vi "Measurement Logic.vi"() -> ()   [LabVIEW 2021, in "audio_acMeasurement.lvlib"]
uses:
  audio_acMeasurement.lvlib
  Measurement Configuration.ctl
  <vilib>/MeasurementLink/MeasurementLink Measurement Server/Classes/MeasurementContext/MeasurementContext.lvclass
  Measurement Results.ctl
  <vilib>/PDM Acquisition Toolkit/host/Classes/Tasks/PCM Input/Controls/DVR PCM Input Task.ctl
  <vilib>/PDM Acquisition Toolkit/host/Classes/Tasks/PCM Input/PCM Input Task.lvclass
  shared/controls/Protocol settings.ctl
  <vilib>/DAQmx/create/channels.llb/DAQmx Create Channel (AO-Voltage-Basic).vi
  <vilib>/DAQmx/configure/timing.llb/DAQmx Timing (Sample Clock).vi
  <vilib>/DAQmx/create/channels.llb/DAQmx Create Channel (AO-FuncGen).vi
  <vilib>/PDM Acquisition Toolkit/host/API/Public/Start/Start PCM Input Task.vi
  <vilib>/PDM Acquisition Toolkit/host/API/Public/Read/Read PCM Input Waveform.vi
  <vilib>/PDM Acquisition Toolkit/host/API/Public/Clear/Clear PCM Input Task.vi
  <resource>/objmgr/daqmx.rc
  <vilib>/PDM Acquisition Toolkit/host/API/PDM Acquisition Toolkit.lvlib
panel:
  out "Measurement Results":T1
  out "Measurement Context out":refnum<class "MeasurementContext.lvclass">
  in  "Measurement Context":refnum<class "MeasurementContext.lvclass">
  in  "Measurement Configuration":T2={"Band start"=20.0, "Band stop"=20000.0, "Weighting filter"=0, "Full scale range"=3.16, "Channel name"="0L", "Analog source resource name"="", "Frequency"=1000.0, "Amplitude"=1.0, "Protocol capture resource name"="", "Data line"=0, "Channel"=0, "Clock rate"=12288000, "Number of words"=19200, "Sensitivity"=0.34762} {"Data line" format="%#.0f"}
  out "error out":errorcluster
  in  "error in":errorcluster
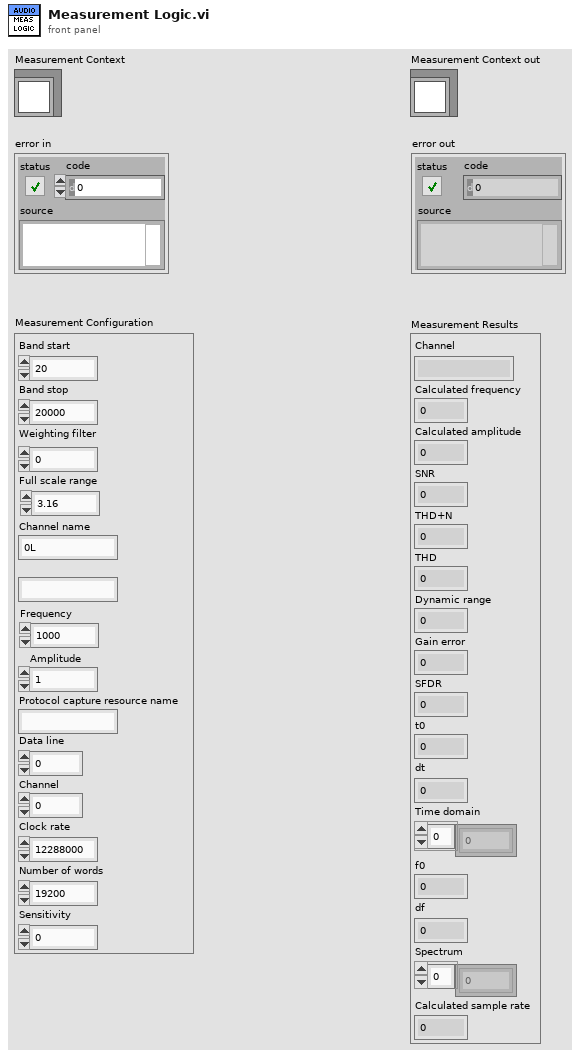
[diagram p1: front panel]
types:
  T1 = typedef "audio_acMeasurement.lvlib/Measurement Results.ctl" = cluster{"Channel":string, "Calculated frequency":dbl, "Calculated amplitude":dbl, "SNR":dbl, "THD+N":dbl, "THD":dbl, "Dynamic range":dbl, "Gain error":dbl, "SFDR":dbl, "t0":dbl, "dt":dbl, "Time domain":dbl[], "f0":dbl, "df":dbl, "Spectrum":dbl[], "Calculated sample rate":u32}
  T2 = typedef "audio_acMeasurement.lvlib/Measurement Configuration.ctl" = cluster{"Band start":dbl, "Band stop":dbl, "Weighting filter":u16, "Full scale range":dbl, "Channel name":string, "Analog source resource name":string, "Frequency":dbl, "Amplitude":dbl, "Protocol capture resource name":string, "Data line":u16, "Channel":u32, "Clock rate":u32, "Number of words":i32, "Sensitivity":dbl}
  T3 = typedef "PDM Acquisition Class Library.lvlib/PCM Input Task.lvclass/DVR PCM Input Task.ctl" = refnum<data-value>
  T4 = cluster{"DSG Session":refnum<k21>, "PDM task":T3}
  T5 = typedef "Protocol settings.ctl" = cluster{"Protocol capture resource name":string, "Data line":u16, "Channel":u32, "Clock rate":u32, "Number of words":i32, "Sensitivity":dbl, "Frame Sync Edge for Channel 0":enum16{"Rising", "Falling"}, "Channel Count Per Frame":u8, "Channel Length":u16, "Bit Depth":u8, "Channel 0 Offset":u16, "Endianness":enum16{"MSB First", "LSB First"}, "Data Justification":enum16{"Left Justified", "Right Justified"}, "Frame Length":u16, "Frame Sync Pulse Width":u16, "Bit Clock Edge  Sync":enum8{"Rising", "Falling"}}
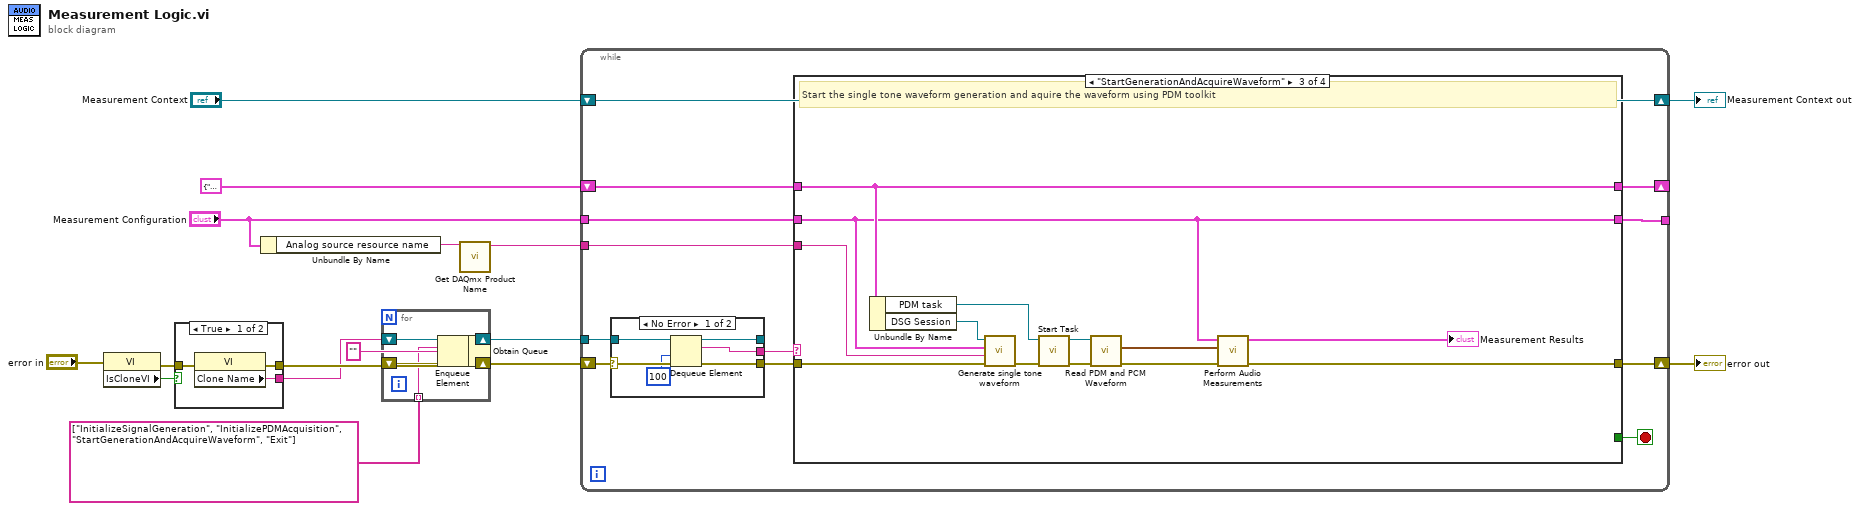
[diagram p0: block diagram]
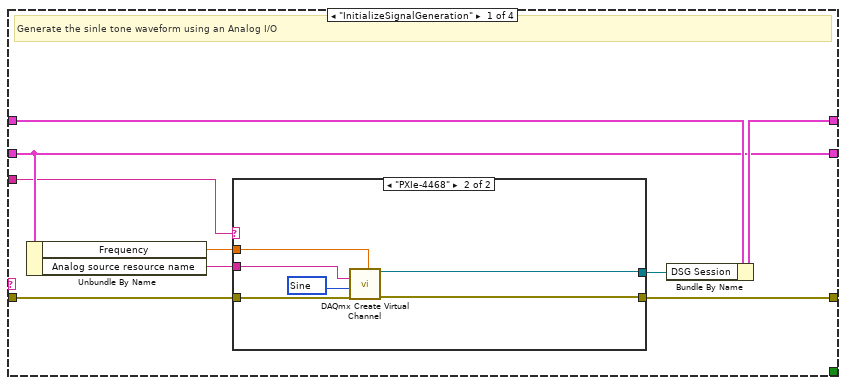
[diagram p2: hidden frame]
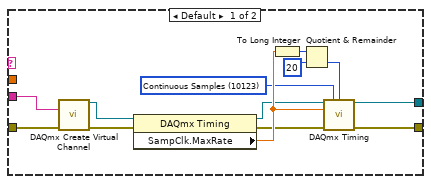
[diagram p3: hidden frame]
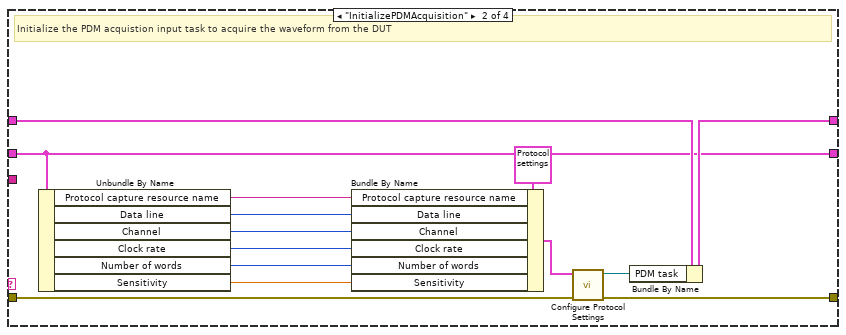
[diagram p4: hidden frame]
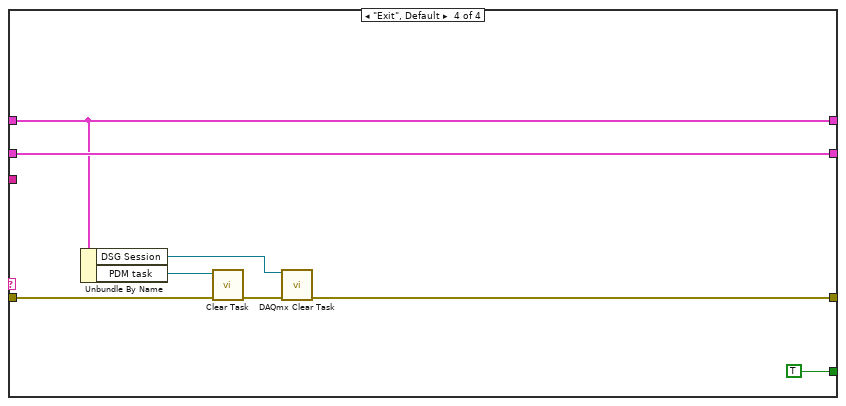
[diagram p5: hidden frame]
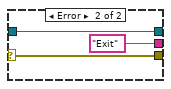
[diagram p6: hidden frame]
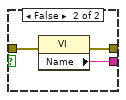
[diagram p7: hidden frame]
diagram:
  n1 = property class="VI"(error in="error in") -> (error out=w15:errorcluster, "IsCloneVI"=w16:bool)  [unwired: 1 in, 1 out]
  n2 = case shown="True" w16 {
    tunnel: [w21 w24] -> w14
    tunnel: [w20 w23] -> w13
    tunnel: w15 -> [w19 w22]
    frame True {
      n3 = property class="VI"(error in=w19) -> (error out=w21:errorcluster, "Clone Name"=w20:string)  [unwired: 1 in, 1 out]
    }
    frame False {
      n4 = property class="VI"(error in=w22) -> (error out=w24:errorcluster, "Name"=w23:string)  [unwired: 1 in, 1 out]
    }
  }
  n5 = Unbundle By Name("Measurement Configuration") -> ("Analog source resource name"=w5:string)
  n6 = call "Get DAQmx Product Name.vi"("DAQmx resource name"=w5) -> ("DAQmx product type"=w3:string)  [unwired: 10 in]
  n7 = Obtain Queue(name (unnamed)=w13, element data type="", error in (no error)=w14) -> (queue out=w17:refnum<queue>, error out=w12:errorcluster)  [unwired: 2 in, 1 out]
  n8 = for {
    shift-right: [w27] -> w11
    shift-left: w17 -> [w29]
    shift-right: [w26] -> w10
    shift-left: w12 -> [w28]
    tunnel: string[] ["InitializeSignalGeneration", "InitializePDMAcquisition", "StartGenerationAndAcquireWaveform", "Exit"] ("Step sequence") -> [w25] mode=indexing
    n9 = Enqueue Element(queue=w29, element=w25, error in (no error)=w28) -> (queue out=w27:refnum<queue>, error out=w26:errorcluster)  [unwired: 1 in, 1 out]
  }
  n10 = while {
    tunnel: w11 -> [w41]
    shift-right: [w38] -> w1
    shift-left: w10 -> [w37]
    shift-right: [w33] -> w6
    shift-left: "Measurement Context" -> [w33]
    tunnel: "Measurement Configuration" -> [w34]
    tunnel: [w35] -> _
    shift-right: [w31] -> _
    shift-left: T4 {"DSG Session"="", "PDM task"=refnum} -> [w36]
    tunnel: w3 -> [w30]
    stop <- w32 stop-if-true
    n11 = case shown="No Error" w37 {
      selector: w37 -> [w108 w112]
      tunnel: w41 -> [w110 w111]
      tunnel: [w109 "Exit" ("t")] -> w40
      tunnel: [w107 w112] -> w39
      tunnel: [w105 w111] -> _
      frame No Error {
        n12 = Dequeue Element(queue=w110, timeout in ms (-1)=100, error in (no error)=w108) -> (queue out=w105:refnum<queue>, element=w109:string, error out=w107:errorcluster)  [unwired: 1 out]
      }
      frame Error {
      }
    }
    n13 = case shown="\"StartGenerationAndAcquireWaveform\"" w40 {
      tunnel: w39 -> [w49 w75 w92 w103]
      tunnel: [w48 w81 w89 w101] -> w38
      tunnel: w34 -> [w45 w79 w86 w104]
      tunnel: w36 -> [w47 w83 w87 w100]
      tunnel: [w46 w82 w87 w100] -> w31
      tunnel: [w45 w79 w86 w104] -> w35
      tunnel: [_ _ _ TRUE] -> w32
      tunnel: w30 -> [w43 _ w84 _]
      frame "InitializeSignalGeneration" {
        # "Generate the sinle tone waveform using an Analog I/O"
        n14 = Unbundle By Name(w45) -> ("Frequency"=w44:dbl, "Analog source resource name"=w50:string)
        n15 = case shown="\"PXIe-4468\"" w43 {
          tunnel: w50 -> [w63 w67]
          tunnel: w49 -> [w62 w69]
          tunnel: [w61 w68] -> w48
          tunnel: [w51 w64] -> w42
          tunnel: w44 -> [_ w65]
          frame Default {
            w52 = 10123 items=["Finite Samples"=10178, "Continuous Samples"=10123, "Hardware Timed Single Point"=12522] ("sample mode")
            n16 = call-poly <vilib>:"DAQmx Create Virtual Channel.vi"("physical channels"=w63, "error in"=w62) -> ("task out"=w60:refnum<k21>, "error out"=w59:errorcluster)  [unwired: 12 in]
            n17 = property class="DAQmx Timing"(reference=w60, error in=w59) -> (reference out=w55:refnum<k21>, error out=w56:errorcluster, "SampClk.MaxRate"=w57:dbl)
            n18 = To Long Integer(number=w57) -> (32bit integer=w53:i32)
            n19 = Quotient & Remainder(x=w53, y=20) -> (floor(x/y)=w58:i32)  [unwired: 1 out]
            n20 = call-poly <vilib>:"DAQmx Timing.vi"("task/channels in"=w55, "sample mode"=w52, "samples per channel"=w58, "rate"=w57, "error in"=w56) -> ("task out"=w51:refnum<k21>, "error out"=w61:errorcluster)  [unwired: 9 in]
          }
          frame "PXIe-4468" {
            w66 = 14751 items=["Sine"=14751, "Triangle"=14752, "Square"=14753, "Sawtooth"=14754] ("type")
            n21 = call-poly <vilib>:"DAQmx Create Virtual Channel.vi"("frequency"=w65, "physical channels"=w67, "type"=w66, "error in"=w69) -> ("task out"=w64:refnum<k21>, "error out"=w68:errorcluster)  [unwired: 10 in]
          }
        }
        n22 = Bundle By Name(cluster=w47, "DSG Session"=w42) -> (w46:T4)
      }
      frame "InitializePDMAcquisition" {
        # "Initialize the PDM acquistion input task to acquire the waveform from the DUT"
        n23 = Unbundle By Name(w79) -> ("Protocol capture resource name"=w72:string, "Data line"=w71:u16, "Channel"=w70:u32, "Clock rate"=w78:u32, "Number of words"=w77:i32, "Sensitivity"=w76:dbl)
        n24 = Bundle By Name(cluster=T5 {"Protocol capture resource name"="", "Data line"=0, "Channel"=0, "Clock rate"=12288000, "Number of words"=19200, "Sensitivity"=0.34762, "Frame Sync Edge for Channel 0"=enum."Falling", "Channel Count Per Frame"=2, "Channel Length"=32, "Bit Depth"=24, "Channel 0 Offset"=1, "Endianness"=enum."MSB First", "Data Justification"=enum."Left Justified", "Frame Length"=64, "Frame Sync Pulse Width"=32, "Bit Clock Edge  Sync"=enum."Falling"} ("Protocol settings"), "Protocol capture resource name"=w72, "Data line"=w71, "Channel"=w70, "Clock rate"=w78, "Number of words"=w77, "Sensitivity"=w76) -> (w73:T5)
        n25 = call "Configure Protocol Settings.vi"("error in"=w75, "Protocol settings"=w73) -> ("error out"=w81:errorcluster, "PDM task"=w80:T3)  [unwired: 8 in]
        n26 = Bundle By Name(cluster=w83, "PDM task"=w80) -> (w82:T4)
      }
      frame "StartGenerationAndAcquireWaveform" {
        # "Start the single tone waveform generation and aquire the waveform using PDM toolkit"
        n27 = Unbundle By Name(w87) -> ("PDM task"=w93:T3, "DSG Session"=w91:refnum<k21>)
        n28 = call "Generate single tone waveform.vi"("error in"=w92, "DAQmx product type"=w84, "Measurement Configuration"=w86, "DSG task in"=w91) -> ("error out"=w94:errorcluster)  [unwired: 6 in, 1 out]
        n29 = call-poly <vilib>:"Start Task.vi"("error in"=w94, "PCM input task in"=w93) -> ("error out"=w96:errorcluster, "PCM input task out"=w95:T3)  [unwired: 8 in]
        n30 = call-poly <vilib>:"Read PDM and PCM Waveform.vi"("error in"=w96, "PCM input task In"=w95) -> ("error out"=w90:errorcluster, "PCM waveforms"=w88:waveform(dbl)[])  [unwired: 4 in, 4 out]
        n31 = call "Perform Audio Measurements.vi"("Measurement Configuration"=w86, "I2S waveforms"=w88, "error in"=w90) -> ("Measurement Results"=→"Measurement Results":T1, "error out"=w89:errorcluster)  [unwired: 6 in]
      }
      frame "Exit", Default {
        n32 = Unbundle By Name(w100) -> ("DSG Session"=w99:refnum<k21>, "PDM task"=w98:T3)
        n33 = call-poly <vilib>:"Clear Task.vi"("error in"=w103, "PCM input task in"=w98) -> ("error out"=w102:errorcluster)  [unwired: 9 in]
        n34 = call <vilib>:"DAQmx Clear Task.vi"("task in"=w99, "error in"=w102) -> ("error out"=w101:errorcluster)  [unwired: 13 in]
      }
    }
  }
  "error out" <- w1
  "Measurement Context out" <- w6
